vi "make_square.vi"(11 "Refnum in":T1) -> (3 "Refnum out":T1)   [LabVIEW 2024]
uses:
  <vilib>/vision/Image Controls.llb/IMAQ Image.ctl
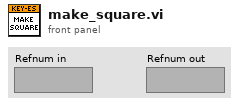
[diagram p1: front panel]
types:
  T1 = typedef "IMAQ Image.ctl" = refnum<image>
  T2 = typedef "Image Type" = u32
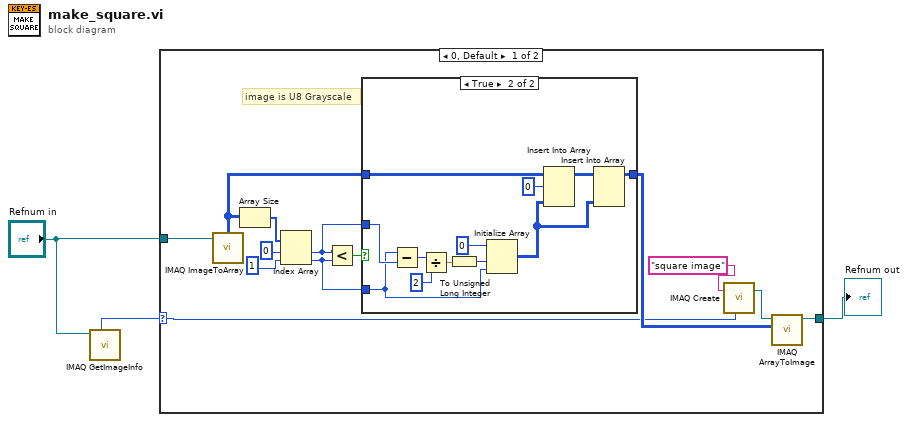
[diagram p0: block diagram]
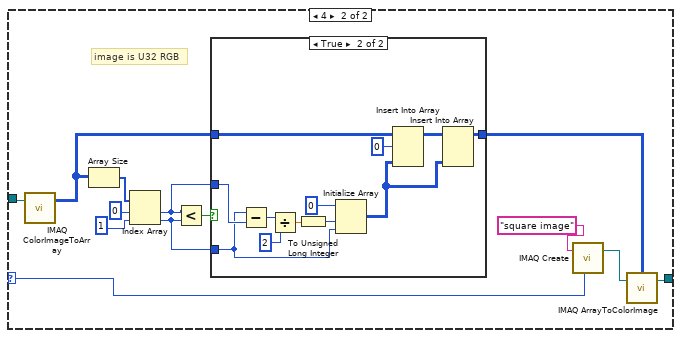
[diagram p3: hidden frame]
diagram:
  n1 = call "IMAQ GetImageInfo"("Image"="Refnum in") -> ("Image Type"=w2:T2)  [unwired: 3 in, 7 out]
  n2 = case shown="0, Default" w2 {
    selector: w2 -> [w4 w33]
    tunnel: [w16 w32] -> w3
    tunnel: "Refnum in" -> [w5 w35]
    frame 0, Default {
      # "image is U8 Grayscale"
      n3 = call "IMAQ ImageToArray"("Image"=w5) -> ("Image Pixels (U8)"=w10:u8[][])  [unwired: 3 in, 4 out]
      n4 = Array Size(array=w10) -> (size(s)=w6:i32[])
      n5 = Index Array(array=w6, index #1=0 ("index"), index #2=1 ("index")) -> (element #1=w11:i32, element #2=w12:i32)
      n6 = Less?(x=w11, y=w12) -> (x < y?=w9:bool)
      n7 = case shown="True" w9 {
        tunnel: w10 -> [w17 w22]
        tunnel: w11 -> [_ w29]
        tunnel: w12 -> [_ w24]
        tunnel: [w17 w18] -> w15
        frame False {
        }
        frame True {
          n8 = Subtract(x=w24, y=w29) -> (x-y=w28:i32)
          n9 = Divide(x=w28, y=2) -> (x/y=w26:dbl)
          n10 = To Unsigned Long Integer(number=w26) -> (unsigned 32bit integer=w25:u32)
          n11 = Initialize Array(u8 0 ("element"), w25, w24) -> (w19:u8[][])
          n12 = Insert Into Array(array=w22, index (row)=0, new element=w19) -> (w20:u8[][])  [unwired: 1 in]
          n13 = Insert Into Array(array=w20, new element=w19) -> (w18:u8[][])  [unwired: 2 in]
        }
      }
      n14 = call "IMAQ Create"("Image Name"="square image", "Image Type"=w4) -> ("New Image"=w13:T1)  [unwired: 3 in, 1 out]
      n15 = call "IMAQ ArrayToImage"("Image Pixels (U8)"=w15, "Image"=w13) -> ("Image Out"=w16:T1)  [unwired: 8 in, 1 out]
    }
    frame 4 {
      # "image is U32 RGB"
      n16 = call "IMAQ ColorImageToArray"("Image"=w35) -> ("Image Pixels (U32)"=w34:u32[][])  [unwired: 3 in, 2 out]
      n17 = Array Size(array=w34) -> (size(s)=w36:i32[])
      n18 = Index Array(array=w36, index #1=0 ("index"), index #2=1 ("index")) -> (element #1=w40:i32, element #2=w41:i32)
      n19 = Less?(x=w40, y=w41) -> (x < y?=w39:bool)
      n20 = case shown="True" w39 {
        tunnel: w34 -> [w43 w48]
        tunnel: w40 -> [_ w55]
        tunnel: w41 -> [_ w50]
        tunnel: [w43 w44] -> w31
        frame False {
        }
        frame True {
          n21 = Subtract(x=w50, y=w55) -> (x-y=w54:i32)
          n22 = Divide(x=w54, y=2) -> (x/y=w52:dbl)
          n23 = To Unsigned Long Integer(number=w52) -> (unsigned 32bit integer=w51:u32)
          n24 = Initialize Array(u8 0 ("element"), w51, w50) -> (w45:u8[][])
          n25 = Insert Into Array(array=w48, index (row)=0, new element=w45) -> (w46:u32[][])  [unwired: 1 in]
          n26 = Insert Into Array(array=w46, new element=w45) -> (w44:u32[][])  [unwired: 2 in]
        }
      }
      n27 = call "IMAQ Create"("Image Name"="square image", "Image Type"=w33) -> ("New Image"=w30:T1)  [unwired: 3 in, 1 out]
      n28 = call "IMAQ ArrayToColorImage"("Image Pixels (U32)"=w31, "Image"=w30) -> ("Image Out"=w32:T1)  [unwired: 3 in, 1 out]
    }
  }
  "Refnum out" <- w3
